vi "PH_HamamatsuCamera.PC set Cam Mode.vi"(0 "i ref in":refnum<vi>, 2 "Select Video Mode":u32(ring), 3 "Tip Strip [Empty]":string, 4 "Strings And Values [Empty]":T1, 5 "error in (no error)":errorcluster) -> (14 "i ref out":refnum<vi>, 17 "Video Mode changed?":bool, 19 "error out":errorcluster)   [LabVIEW 2014]
doc: "This VI checks wether the requested and the current camera video mode are the same or not. If not, it saves the requested mode to own attributes and sets the GUI elements. Video Mode changed? is true in this case."
uses:
  PH_HamamatsuCamera.lvlib
  <vilib>/Utility/miscctls.llb/LVStringsAndValuesArrayTypeDef_U32.ctl
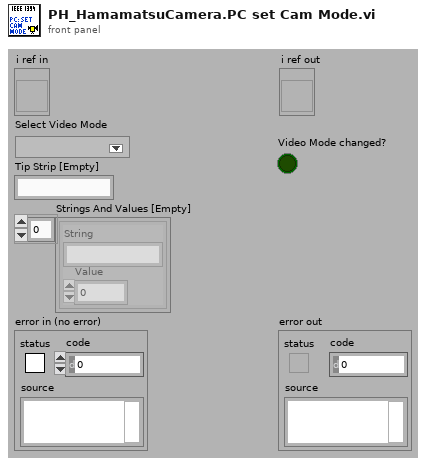
[diagram p1: front panel]
types:
  T1 = typedef "LVStringsAndValuesArrayTypeDef_U32.ctl" = cluster{"String":string, "Value":u32}[]
  T2 = typedef "PH_HamamatsuCamera.lvlib/PH_HamamatsuCamera.i attribute.ctl" = cluster{"Gui Refs":cluster{"Frame Rate":refnum<vi>, "Get Frame Rate":refnum<vi>, "Camera State":refnum<vi>, "Start Cam":refnum<vi>, "Show Image":refnum<vi>, "Get Histogram":refnum<vi>, "Mapping":refnum<vi>, "Histogram":refnum<vi>, "Center Cross":refnum<vi>, "Center of Gravity":refnum<vi>, "Scale Factor [%]":refnum<vi>, "Save Image":refnum<vi>, "Palette":refnum<vi>, "Connect":refnum<vi>, "Camera State Bar":refnum<vi>, "Cam Error":refnum<vi>, "Camera Details":refnum<vi>, "ROI":refnum<vi>, "Set ROI to Maximum":refnum<vi>, "Trigger Parameters":refnum<vi>, "Brightness":refnum<vi>, "Shutter":refnum<vi>, "Gain":refnum<vi>, "Trigger Timeout":refnum<vi>, "Subtract Background":refnum<vi>, "Cam List":refnum<vi>, "Parameters":refnum<vi>, "Trigger Polarity":refnum<vi>, "Trigger Mode":refnum<vi>}, "Cam":cluster{"State":T3, "Restart":bool, "Source Notifier":refnum<notifier>, "Handle":i32, "Details":cluster{"Model":string, "Camera ID":string, "Firmware":string}, "Error":errorcluster, "Buffer Info":cluster{"height":u32, "width":u32, "datatype":u32}}, "Images":cluster{"CamI16":T4, "OperationI16":T4, "PSDB I16":T4}, "Window Image":cluster{"Indicate Image":bool, "Window No.":i32, "Scale Facor":dbl, "Center Cross":bool, "Subtract Backgr":bool, "CoG":bool, "Color Palette":cluster{"Red":u8, "Green":u8, "Blue":u8}[], "Image On":bool}, "Default Prdc Int":i32, "Performance":cluster{"on":bool, "Timestamp Last Frame":i32}, "Histogram":cluster{"on":bool, "Mapping":bool}, "Save Image":cluster{"Save":bool, "File refnum":refnum<file>}, "Setting Service ID":i32, "GUI Manager Path":string, "Screen":cluster{"x-resolution":i16, "y-resolution":i16}, "Image Position Path":string, "H Offset":cluster{"Value":i32, "Minimum":i32, "Maximum":i32, "Increment":i32}, "V Offset":cluster{"Value":i32, "Minimum":i32, "Maximum":i32, "Increment":i32}, "H Width":cluster{"Value":i32, "Minimum":i32, "Maximum":i32, "Increment":i32}, "V Width":cluster{"Value":i32, "Minimum":i32, "Maximum":i32, "Increment":i32}, "Trigger Parameters":cluster{"Mode":u32, "Polarity":u32, "Times":u32, "Delay":dbl}, "Trigger Timeout":u32, "Parameters":T5[], "Cam Setting Parameters":cluster{"Brightness":string, "Shutter":string, "Gain":string}}
  T3 = typedef "Device State.ctl" = i32
  T4 = typedef "IMAQ Image.ctl" = refnum<image>
  T5 = typedef "PH_HamamatsuCamera.lvlib/PH_HamamatsuCamera.Parameter Set.ctl" = cluster{"Name":string, "Value":dbl, "Range":cluster{"min":dbl, "max":dbl, "step":dbl}}
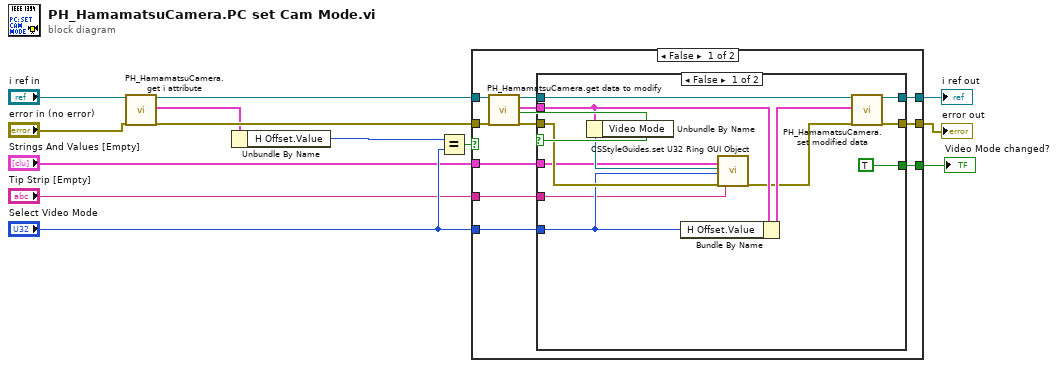
[diagram p0: block diagram]
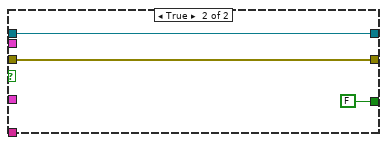
[diagram p2: hidden frame]
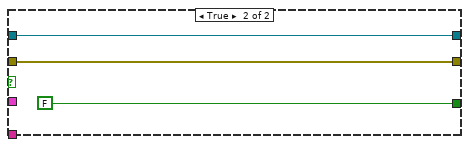
[diagram p3: hidden frame]
diagram:
  n1 = call "PH_HamamatsuCamera.get i attribute.vi"("i ref in"="i ref in", "error in (no error)"="error in (no error)") -> ("i ref out"=w9:refnum<vi>, "i attribute"=w4:T2, "error out"=w7:errorcluster)  [unwired: 15 in]
  n2 = Unbundle By Name(w4) -> ("H Offset.Value"=w11:i32)
  n3 = Equal?(x=w11, y="Select Video Mode") -> (x = y?=w10:bool)
  n4 = case shown="False" w10 {
    tunnel: w9 -> [w25 w42]
    tunnel: w7 -> [w24 w43]
    tunnel: [w22 w42] -> w8
    tunnel: [w20 w43] -> w6
    tunnel: [w17 FALSE] -> w5
    tunnel: "Select Video Mode" -> [w16 _]
    tunnel: "Tip Strip [Empty]" -> [w15 _]
    tunnel: "Strings And Values [Empty]" -> [w14 _]
    frame False {
      n5 = call "PH_HamamatsuCamera.get data to modify.vi"("i ref in"=w25, "error in (no error)"=w24) -> ("i ref out"=w23:refnum<vi>, "i attribute"=w19:T2, "timed out"=w18:bool, "error out"=w21:errorcluster)  [unwired: 14 in]
      n6 = case shown="False" w18 {
        tunnel: w23 -> [w37 w40]
        tunnel: [w36 w40] -> w22
        tunnel: w21 -> [w30 w39]
        tunnel: [w35 w39] -> w20
        tunnel: w19 -> [w33 _]
        tunnel: [TRUE FALSE] -> w17
        tunnel: w16 -> [w28 _]
        tunnel: w15 -> [w27 _]
        tunnel: w14 -> [w26 _]
        frame False {
          n7 = Unbundle By Name(w33) -> ("Video Mode"=w31:refnum<vi>)
          n8 = Bundle By Name(cluster=w33, "H Offset.Value"=w28) -> (w34:T2)
          n9 = call "CSStyleGuides.set U32 Ring GUI Object.vi"("Strings And Values [Empty]"=w26, "Ring Ref"=w31, "Value"=w28, "error in (no error)"=w30, "Tip Strip [Empty]"=w27) -> ("error out"=w29:errorcluster)  [unwired: 14 in]
          n10 = call "PH_HamamatsuCamera.set modified data.vi"("i ref in"=w37, "i attribute"=w34, "error in (no error)"=w29) -> ("i ref out"=w36:refnum<vi>, "error out"=w35:errorcluster)  [unwired: 15 in]
        }
        frame True {
        }
      }
    }
    frame True {
    }
  }
  "error out" <- w6
  "i ref out" <- w8
  "Video Mode changed?" <- w5
